vi "lockin - replace AO Sweep Indicator.vi"(8 "error in (no error)":errorcluster, 10 "Channels: AO.Sweep?":bool[](array[boolean]), 11 "Lockin.DAQ":refnum<class "Lockin.DAQ.lvclass">) -> (0 "error out":errorcluster, 3 "Lockin.DAQ out":refnum<class "Lockin.DAQ.lvclass">)   [LabVIEW 2016, in "Lockin.DAQ.lvclass"]
uses:
  Lockin.DAQ.lvclass
  Lockin.DAQ.lvclass/Lockin.DAQ.ctl
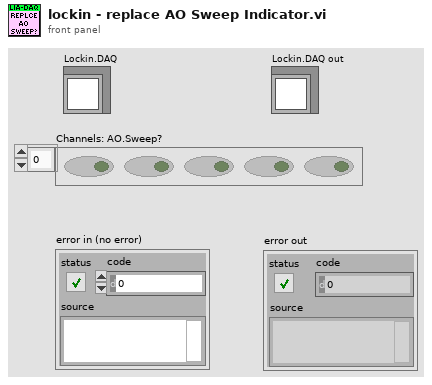
[diagram p1: front panel]
types:
  T1 = typedef "Lockin.DAQ.lvclass/AO-cluster.ctl" = T2[]
  T2 = typedef "Instrument.Lockin.UI.lvclass/AO Channel--Cluster.ctl" = cluster{"Enable?":bool, "Channel":i32, "Amplitude":dbl, "Offset":dbl, "Frequency":dbl, "Phase":dbl, "Function":T3, "Sweeping?":bool}
  T3 = typedef "Lockin.DAQ.lvclass/Function-enum.ctl" = enum16{"Sine", "Triangle", "Square"}
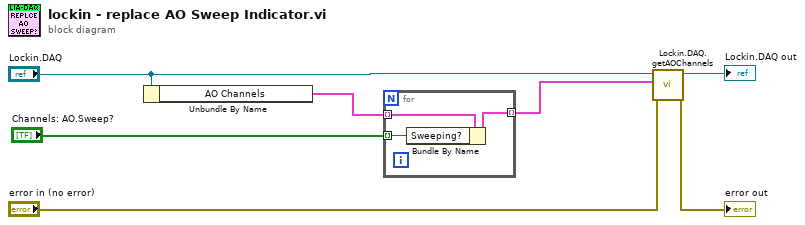
[diagram p0: block diagram]
diagram:
  n1 = Unbundle By Name("Lockin.DAQ") -> ("AO Channels"=w3:T1)
  n2 = for {
    tunnel: w3 -> [w10] mode=indexing
    tunnel: "Channels: AO.Sweep?" -> [w9] mode=indexing
    tunnel: [w8] -> w1 mode=indexing
    n3 = Bundle By Name(cluster=w10, "Sweeping?"=w9) -> (w8:T2)
  }
  n4 = call "Lockin.DAQ.getAOChannels.vi"("error in (no error)"="error in (no error)", "Channels: AO"=w1, "Lockin.DAQ"="Lockin.DAQ") -> ("error out"=→"error out":errorcluster, "Lockin.DAQ"=→"Lockin.DAQ out":refnum<class "Lockin.DAQ.lvclass">)  [unwired: 7 in]
